vi "UnregisterPublisher.vi"(7 "Topic Name":string, 8 "error in (no error)":errorcluster, 11 "Message Broker in":refnum<class "Message Broker.lvclass">) -> (0 "error out":errorcluster, 3 "Message Broker out":refnum<class "Message Broker.lvclass">)   [LabVIEW 2016, in "Stream Mediator.lvlib" / "Message Broker.lvclass"]
doc: "--\nCopyright © 2017 Composed SystemsI All rights reserved.\n\nAuthor: Jon McBee <jon.mcbee@composed.io>\n\nThis library is provided \"AS IS\" ,WITHOUT WARRANTIES OR\nCONDITIONS OF ANY KIND, either express or implied.\n\nComposed Systems -- composed.io\n\nStream 0.0.1.1\nJon McBee - Composed Systems\nCopyright (c) 2017, Composed Systems"
uses:
  <userlib>/Composed Systems/Stream/Mediator/Classes/Message Broker/Message Broker.lvclass
  <userlib>/Composed Systems/Stream/Mediator/Classes/Message Broker/Message Broker.lvclass/Message Broker.ctl
  <userlib>/Composed Systems/Stream/Mediator/Classes/Topic Actor Look Up Table/Topic Actor Look Up Table.lvclass
  <userlib>/Composed Systems/Stream/Mediator/Classes/Topic Actor Descriptor/Topic Actor Descriptor.lvclass
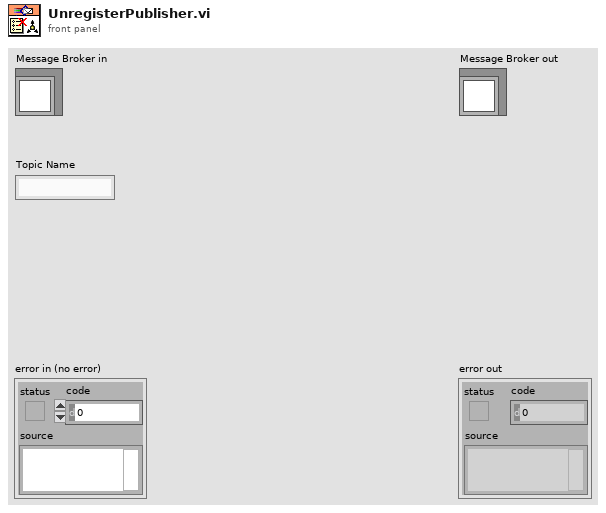
[diagram p1: front panel]
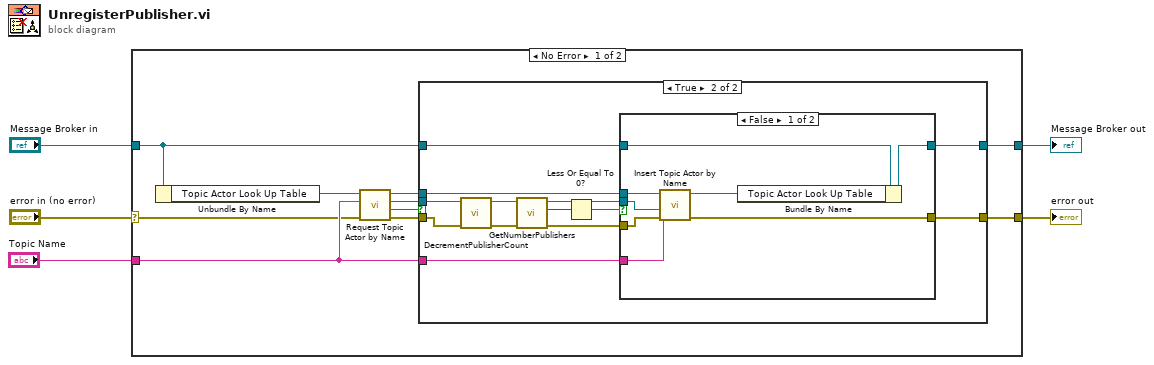
[diagram p0: block diagram]
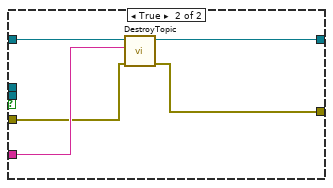
[diagram p3: hidden frame]
diagram:
  n1 = case shown="No Error" "error in (no error)" {
    selector: "error in (no error)" -> [w7 w45]
    tunnel: [w6 w45] -> w4
    tunnel: [w11 w44] -> w2
    tunnel: "Message Broker in" -> [w12 w44]
    tunnel: "Topic Name" -> [w9 _]
    frame No Error {
      n2 = Unbundle By Name(w12) -> ("Topic Actor Look Up Table"=w15:refnum<class "Topic Actor Look Up Table.lvclass">)
      n3 = call <userlib>:"Request Topic Actor by Name.vi"("error in (no error)"=w7, "Topic Actor"=w9, "Topic Actor Look Up Table in"=w15) -> ("error out"=w8:errorcluster, "Found?"=w14:bool, "Topic Actor Descriptor"=w10:refnum<class "Topic Actor Descriptor.lvclass">, "Topic Actor Look Up Table out"=w13:refnum<class "Topic Actor Look Up Table.lvclass">)  [unwired: 5 in]
      n4 = case shown="True" w14 {
        tunnel: w13 -> [_ w25]
        tunnel: [w17 w23] -> w11
        tunnel: w12 -> [w17 w26]
        tunnel: w10 -> [_ w30]
        tunnel: w9 -> [_ w24]
        tunnel: w8 -> [w16 w22]
        tunnel: [w16 w19] -> w6
        frame False {
        }
        frame True {
          n5 = call <userlib>:"DecrementPublisherCount.vi"("error in (no error)"=w22, "Topic Actor Descriptor in"=w30) -> ("error out"=w21:errorcluster, "Topic Actor Descriptor out"=w29:refnum<class "Topic Actor Descriptor.lvclass">)  [unwired: 8 in]
          n6 = call <userlib>:"GetNumberPublishers.vi"("error in (no error)"=w21, "Topic Actor Descriptor in"=w29) -> ("error out"=w20:errorcluster, "N Publishers"=w28:u32, "Topic Actor Descriptor out"=w18:refnum<class "Topic Actor Descriptor.lvclass">)  [unwired: 7 in]
          n7 = Less Or Equal To 0?(x=w28) -> (x <= 0?=w27:bool)
          n8 = case shown="False" w27 {
            tunnel: [w32 w42] -> w23
            tunnel: w26 -> [w38 w43]
            tunnel: w25 -> [w37 _]
            tunnel: w24 -> [w34 w41]
            tunnel: w20 -> [w36 w40]
            tunnel: [w35 w39] -> w19
            tunnel: w18 -> [w33 _]
            frame False {
              n9 = call <userlib>:"Insert Topic Actor by Name.vi"("error in (no error)"=w36, "Topic Actor Descriptor"=w33, "Topic Actor"=w34, "Topic Actor Look Up Table in"=w37) -> ("error out"=w35:errorcluster, "Topic Actor Look Up Table out"=w31:refnum<class "Topic Actor Look Up Table.lvclass">)  [unwired: 5 in, 1 out]
              n10 = Bundle By Name(cluster=w38, "Topic Actor Look Up Table"=w31) -> (w32:refnum<class "Message Broker.lvclass">)
            }
            frame True {
              n11 = call <userlib>:"DestroyTopic.vi"("error in (no error)"=w40, "Topic Actor"=w41, "Message Broker in"=w43) -> ("error out"=w39:errorcluster, "Message Broker out"=w42:refnum<class "Message Broker.lvclass">)  [unwired: 6 in, 1 out]
            }
          }
        }
      }
    }
    frame Error {
    }
  }
  "error out" <- w4
  "Message Broker out" <- w2
